vi "Read all Results.vi"(8 "error in (no error)":errorcluster, 11 "Data Value Reference in":refnum<data-value>) -> (0 "error out":errorcluster, 1 "Surveys Count":i32, 2 "Array":cluster{" Average":dbl, T1}[](array[cluster]), 3 "Data Value Reference out":refnum<data-value>)   [LabVIEW 2016, in "Data Operations.lvlib"]
uses:
  Data Operations.lvlib
  Private Controls/Survey Results Enum.ctl
  Private Controls/Data Raw.ctl
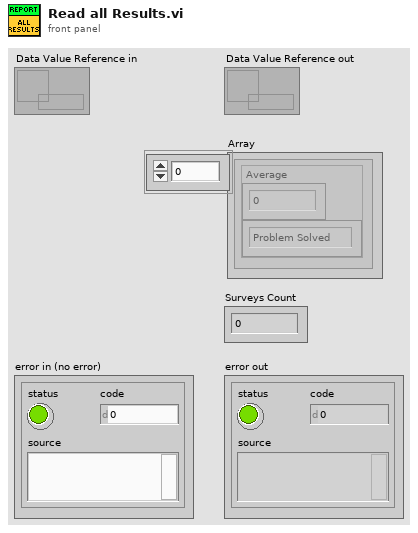
[diagram p1: front panel]
types:
  T1 = typedef "Data Operations.lvlib/Survey Results Enum.ctl" = enum16{"Problem Solved", "Resolution Time", "Total Satisfaction", "Courtesy", "Response Time"}
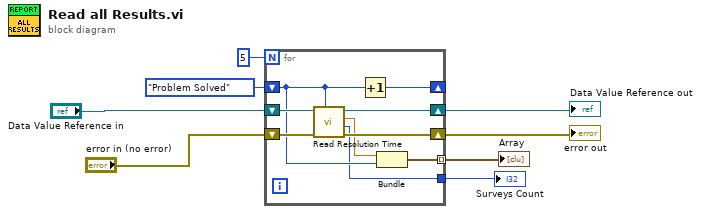
[diagram p0: block diagram]
diagram:
  n1 = for {
    N: 5 -> [_]
    shift-right: [w14] -> w4
    shift-left: "Data Value Reference in" -> [w17]
    shift-right: [w15] -> w3
    shift-left: "error in (no error)" -> [w16]
    shift-right: [w13] -> _
    shift-left: Survey_Results_Enum."Problem Solved" -> [w11]
    tunnel: [w10] -> w7 mode=indexing
    tunnel: [w9] -> w8
    n2 = call "Read Resolution Time.vi"("Enum"=w11, "Error In"=w16, "DVR IN"=w17) -> ("Error Out"=w15:errorcluster, "Surveys Count"=w9:i32, "Average"=w12:dbl, "Data Value Reference out"=w14:refnum<data-value>)  [unwired: 5 in]
    n3 = Increment(x=w11) -> (x+1=w13:T1)
    n4 = Bundle("Average"=w12, w11) -> (w10:cluster{" Average":dbl, T1})  [unwired: 1 in]
  }
  "Surveys Count" <- w8
  "Array" <- w7
  "Data Value Reference out" <- w4
  "error out" <- w3
